vi "create glyph manager.vi"(8 "error in":errorcluster, 11 "tree ref (for default symbols)":refnum<vi>) -> (0 "error out":errorcluster, 3 "glyph manager":T1)   [LabVIEW 2013, in "glyph manager.lvlib"]
uses:
  glyph manager.lvlib
  glyph manager.ctl
  <vilib>/picture/picture.llb/imagedata.ctl
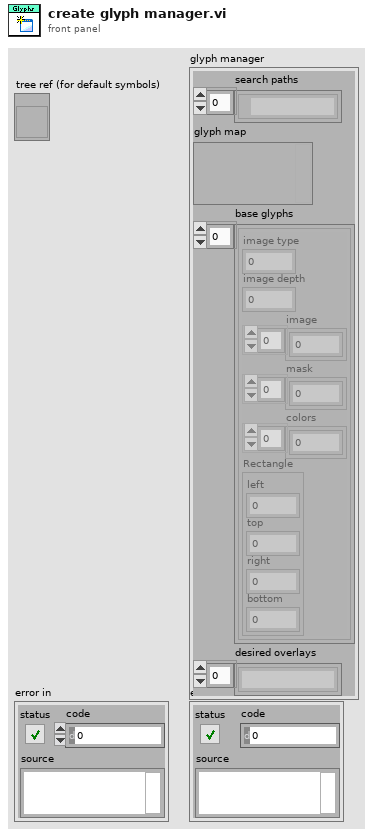
[diagram p1: front panel]
types:
  T1 = typedef "glyph manager.lvlib/glyph manager.ctl" = cluster{"search paths":path[], "glyph map":variant, "base glyphs":T2[], "desired overlays":string[]}
  T2 = typedef "imagedata.ctl" = cluster{"image type":i32, "image depth":i32, "image":u8[], "mask":u8[], "colors":u32[], "Rectangle":cluster{"left":i16, "top":i16, "right":i16, "bottom":i16}}
  T3 = cluster{"image type":i32, "image depth":i32, "image":u8[], "mask":u8[], "colors":u32[], "Rectangle":cluster{"left":i16, "top":i16, "right":i16, "bottom":i16}}[]
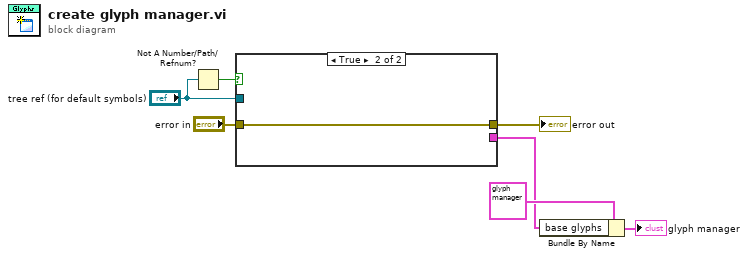
[diagram p0: block diagram]
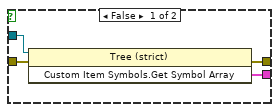
[diagram p2: hidden frame]
diagram:
  n1 = Not A Number/Path/Refnum?(number/path/refnum="tree ref (for default symbols)") -> (NaN/Path/Refnum?=w1:bool)
  n2 = case shown="True" w1 {
    tunnel: [w11 _] -> w6
    tunnel: "error in" -> [w10 w12]
    tunnel: [w9 w12] -> w4
    tunnel: "tree ref (for default symbols)" -> [w8 _]
    frame False {
      n3 = invoke class="Tree (strict)" method="Custom Item Symbols.Get Symbol Array"(reference=w8, error in=w10) -> (error out=w9:errorcluster, "Custom Glyphs:Get Glyph Array"=w11:T3)  [unwired: 1 in, 1 out]
    }
    frame True {
    }
  }
  "error out" <- w4
  n4 = Bundle By Name(cluster=T1 {"search paths"=[], "glyph map"=variant, "base glyphs"=[], "desired overlays"=[]} ("glyph manager"), "base glyphs"=w6) -> (→"glyph manager":T1)
